vi "ByteWrite.vi"(7 "data":u8[](array[numeric]), 8 "error in (no error)":errorcluster, 9 "command":u8, 10 "Serial Settings":T1 {"flow control" items=["None"=0, "XON/XOFF"=1, "RTS/CTS"=2, "DTR/DSR"=4]; "stop bits" items=["1.0"=10, "1.5"=15, "2.0"=20]; "data bits" min=5 max=8 step=1; "baud rate" items=["75"=75, "110"=110, "134"=134, "150"=150, "300"=300, "600"=600, "1200"=1200, "1800"=1800, "2400"=2400, "4800"=4800, "7200"=7200, "9600"=9600, "14400"=14400, "19200"=19200, "28800"=28800, "38400"=38400, "56000"=56000, "57600"=57600, "115200"=115200, "128000"=128000, "230400"=230400]}, 11 "VISA Refnum in":refnum<visa-resource-name>) -> (0 "error out":errorcluster, 2 "Packet Size":u32, 3 "VISA Refnum out":refnum<visa-resource-name>)   [LabVIEW 2019]
uses:
  Design of uP Systems/Serial - Settings.ctl
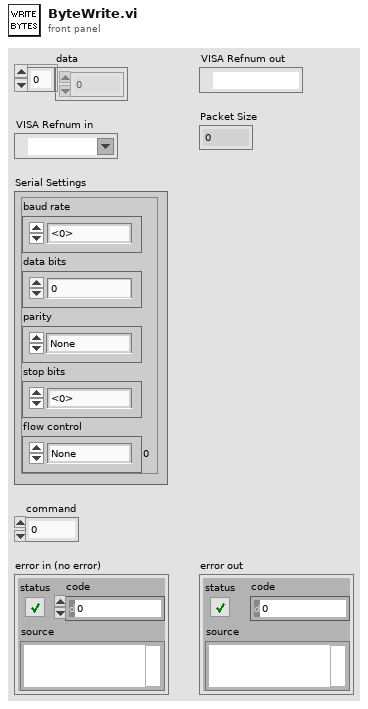
[diagram p1: front panel]
types:
  T1 = typedef "Serial - Settings.ctl" = cluster{"baud rate":u32, "data bits":u16, "parity":enum16{"None", "Odd", "Even", "Mark", "Space"}, "stop bits":u16, "flow control":u16}
  T2 = cluster{"Packet_Size":u8, "command":u8, "buffer":u8[]}
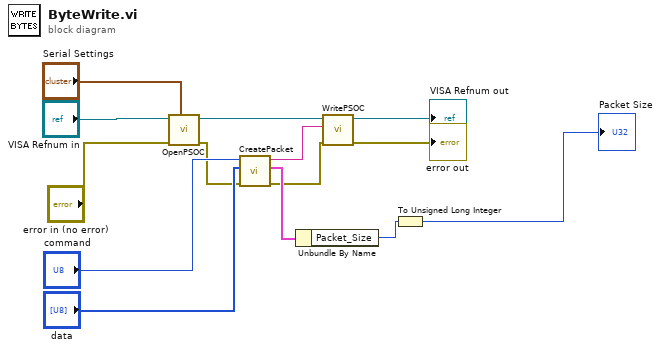
[diagram p0: block diagram]
diagram:
  n1 = call "OpenPSOC.vi"("Serial Settings"="Serial Settings", "error in"="error in (no error)", "VISA resource name"="VISA Refnum in") -> ("error out"=w4:errorcluster, "VISA resource name out"=w6:refnum<visa-resource-name>)  [unwired: 7 in]
  n2 = call "CreatePacket.vi"("error in"=w4, "data"="data", "command"="command") -> ("error out"=w5:errorcluster, "output cluster"=w8:T2, "Command String"=w14:string)  [unwired: 6 in]
  n3 = Unbundle By Name(w8) -> ("Packet_Size"=w9:u8)
  n4 = call "WritePSOC.vi"("error in"=w5, "write buffer"=w14, "VISA resource name"=w6) -> ("error out"=→"error out":errorcluster, "VISA resource name out"=→"VISA Refnum out":refnum<visa-resource-name>)  [unwired: 5 in, 1 out]
  n5 = To Unsigned Long Integer(number=w9) -> (unsigned 32bit integer=→"Packet Size":u32)
